vi "Starter Kit 2.0 Custom RT Host.vi"() -> ()   [LabVIEW 2021]
doc: "This VI shows how to use hardware abstracted sensor drivers with a custom FPGA VI to control a Starter Kit robot. This VI runs on the RT host. The main FPGA VI must be compiled before this host VI can be run."
uses:
  <vilib>/rvi/interface/nirviOpenFPGA/nirviOpenFPGA.xnode
  <instrlib>/DC Motor Controller/HAIOL/DC Motor Controller.lvclass
  <vilib>/rvi/interface/nirviCloseFPGA/nirviCloseFPGA.xnode
  <vilib>/rvi/interface/nirviReadWriteControl/nirviReadWriteControl.xnode
  <vilib>/robotics/Utilities/RPM to Radians per Second (Scalar).vi
  <vilib>/robotics/Utilities/Radians per Second to RPM (Scalar).vi
  <vilib>/Utility/AngleManip/NI_AngleManipulation.lvlib
  <vilib>/rvi/interface/Simulation/niFpgaSimulationCallBeginRW.vi
  <vilib>/rvi/errors/niLvFpgaAdjustHostInterfaceError.vi
  <vilib>/Platform/TimedLoop/XDataNode/XDataNode.xnode
  <vilib>/Platform/TimedLoop/XDataNode/nitl_modes.ctl
  <vilib>/Platform/TimedLoop/XDataNode/XDNodeRunTimeDep.lvlib
  <vilib>/Platform/TimedLoop/XDataNode/wakeup.ctl
  <vilib>/Platform/TimedLoop/XDataNode/timing_clust.ctl
  <vilib>/Utility/error.llb/Error Cluster From Error Code.vi
  <instrlib>/Hitec HS400 Series/HAIOL/Hitec HS400 Series.lvclass
  <instrlib>/Parallax PING)))/HAIOL/Parallax PING))).lvclass
  <vilib>/Utility/AngleManip/Degrees to Radians (Scalar DBL).vi
  FPGA Bitfiles/MintaDaNIrobotho_FPGATarget_StarterKit2.0Cus_29373616.lvbitx
  NiFpgaLv.dll
  <vilib>/FPGAPlugInAG/Dynamic/niLvFpga_Close_Dynamic.vi
  <vilib>/FPGAPlugInAG/sbRIO-9632/niLvFpga_Open_sbRIO-9632.vi
  <vilib>/rvi/interface/common/dynamic/niFpgaDynamicAddResources.vi
panel:
  out "P(k|k)":dbl
  out "rho(k|k)":dbl
  out "theta error":dbl
  out "theta(i+1)":dbl
  out "y(i+1)":dbl
  out "x(i+1)":dbl
  out "theta(i)":dbl
  out "y(i)":dbl
  out "x(i)":dbl
  out "right wheel dist":dbl
  out "left wheel dist":dbl
  out "CMPS03 angle":sgl(knob) scale=0.0..360.0 scale format="%#_4f"
  in  "stop":bool
  in  "Common":dbl(slide) min=-100.0 max=100.0 step=4.0 scale=-100.0..100.0
  in  "Diff":dbl(slide) min=-100.0 max=100.0 step=4.0 scale=-100.0..100.0
  out "ccw motor velocities":cluster{"Left":dbl, dbl, "Right":dbl, dbl}(graph)
  in  "sensor motor angle":dbl(slide) caption="Sensor Motor Angle (degrees)" scale=90.0..-90.0
  out "PING))) Sensor Distance (m)":dbl(graph)
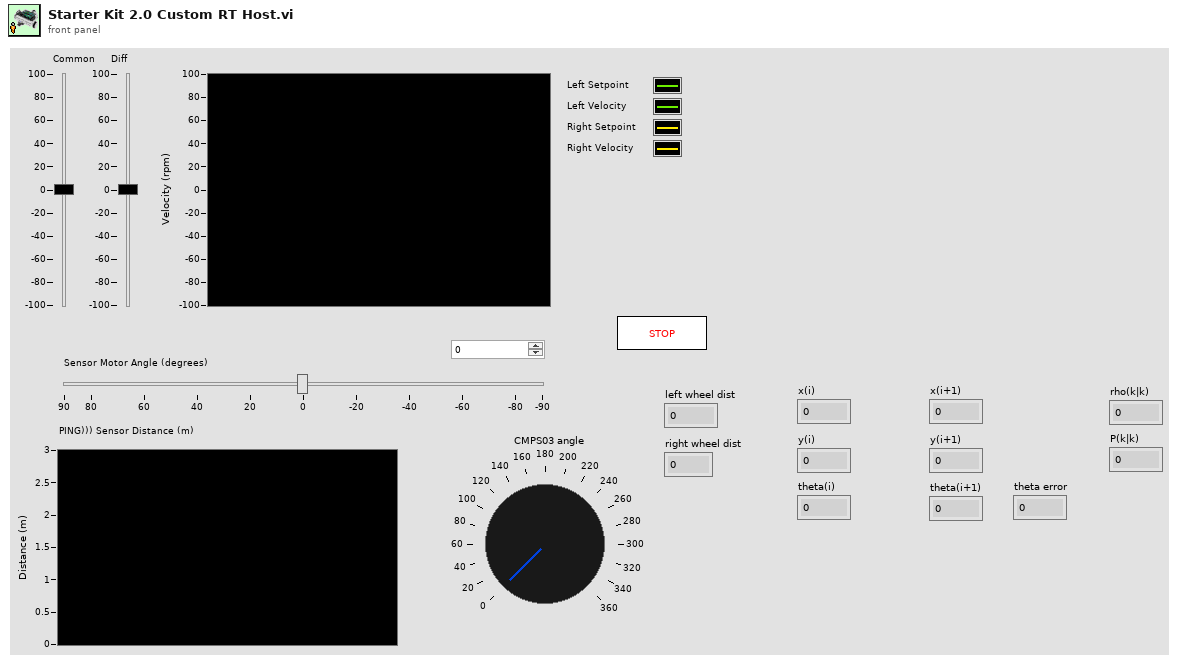
[diagram p1: front panel]
types:
  T1 = typedef "XDNodeRunTimeDep.lvlib/timing_clust.ctl" = cluster{"Expected End [f-1]":u64, "Actual End [f-1]":u64, "Finished Late? [f-1]":bool, "Expected End [i-1]":u64, "Actual End [i-1]":u64, "Finished Late? [i-1]":bool, "Expected Start [i]":u64, "Actual Start [i]":u64, "Expected Start [f]":u64, "Actual Start [f]":u64, "Source Name":string, "Structure Name":string, "Period":i64, "Deadline":i64, "Offset":i64, "Start":i64, "Priority":i32, "Timeout":i32, "Mode":T2, "Wakeup Reason":T3, "Error":errorcluster, "Source Type":string, "Secondary Source Type":string, "Global End Time":u64, "Global Start Time":u64, "Frame Duration":u64, "Iteration Duration":u64, "Assigned CPU":i32, "I/O Scan Engine Mode":u32}
  T2 = typedef "XDNodeRunTimeDep.lvlib/nitl_modes.ctl" = enum32{"No Change", "Process missed periods, maintain original phase", "Discard missed periods, maintain original phase", "Process missed periods, ignore original phase", "Discard missed periods, ignore original phase"}
  T3 = typedef "XDNodeRunTimeDep.lvlib/wakeup.ctl" = enum32{"Normal", "Aborted", "Asynchronous wakeup", "Timing source error", "Timed loop error", "Timeout"}
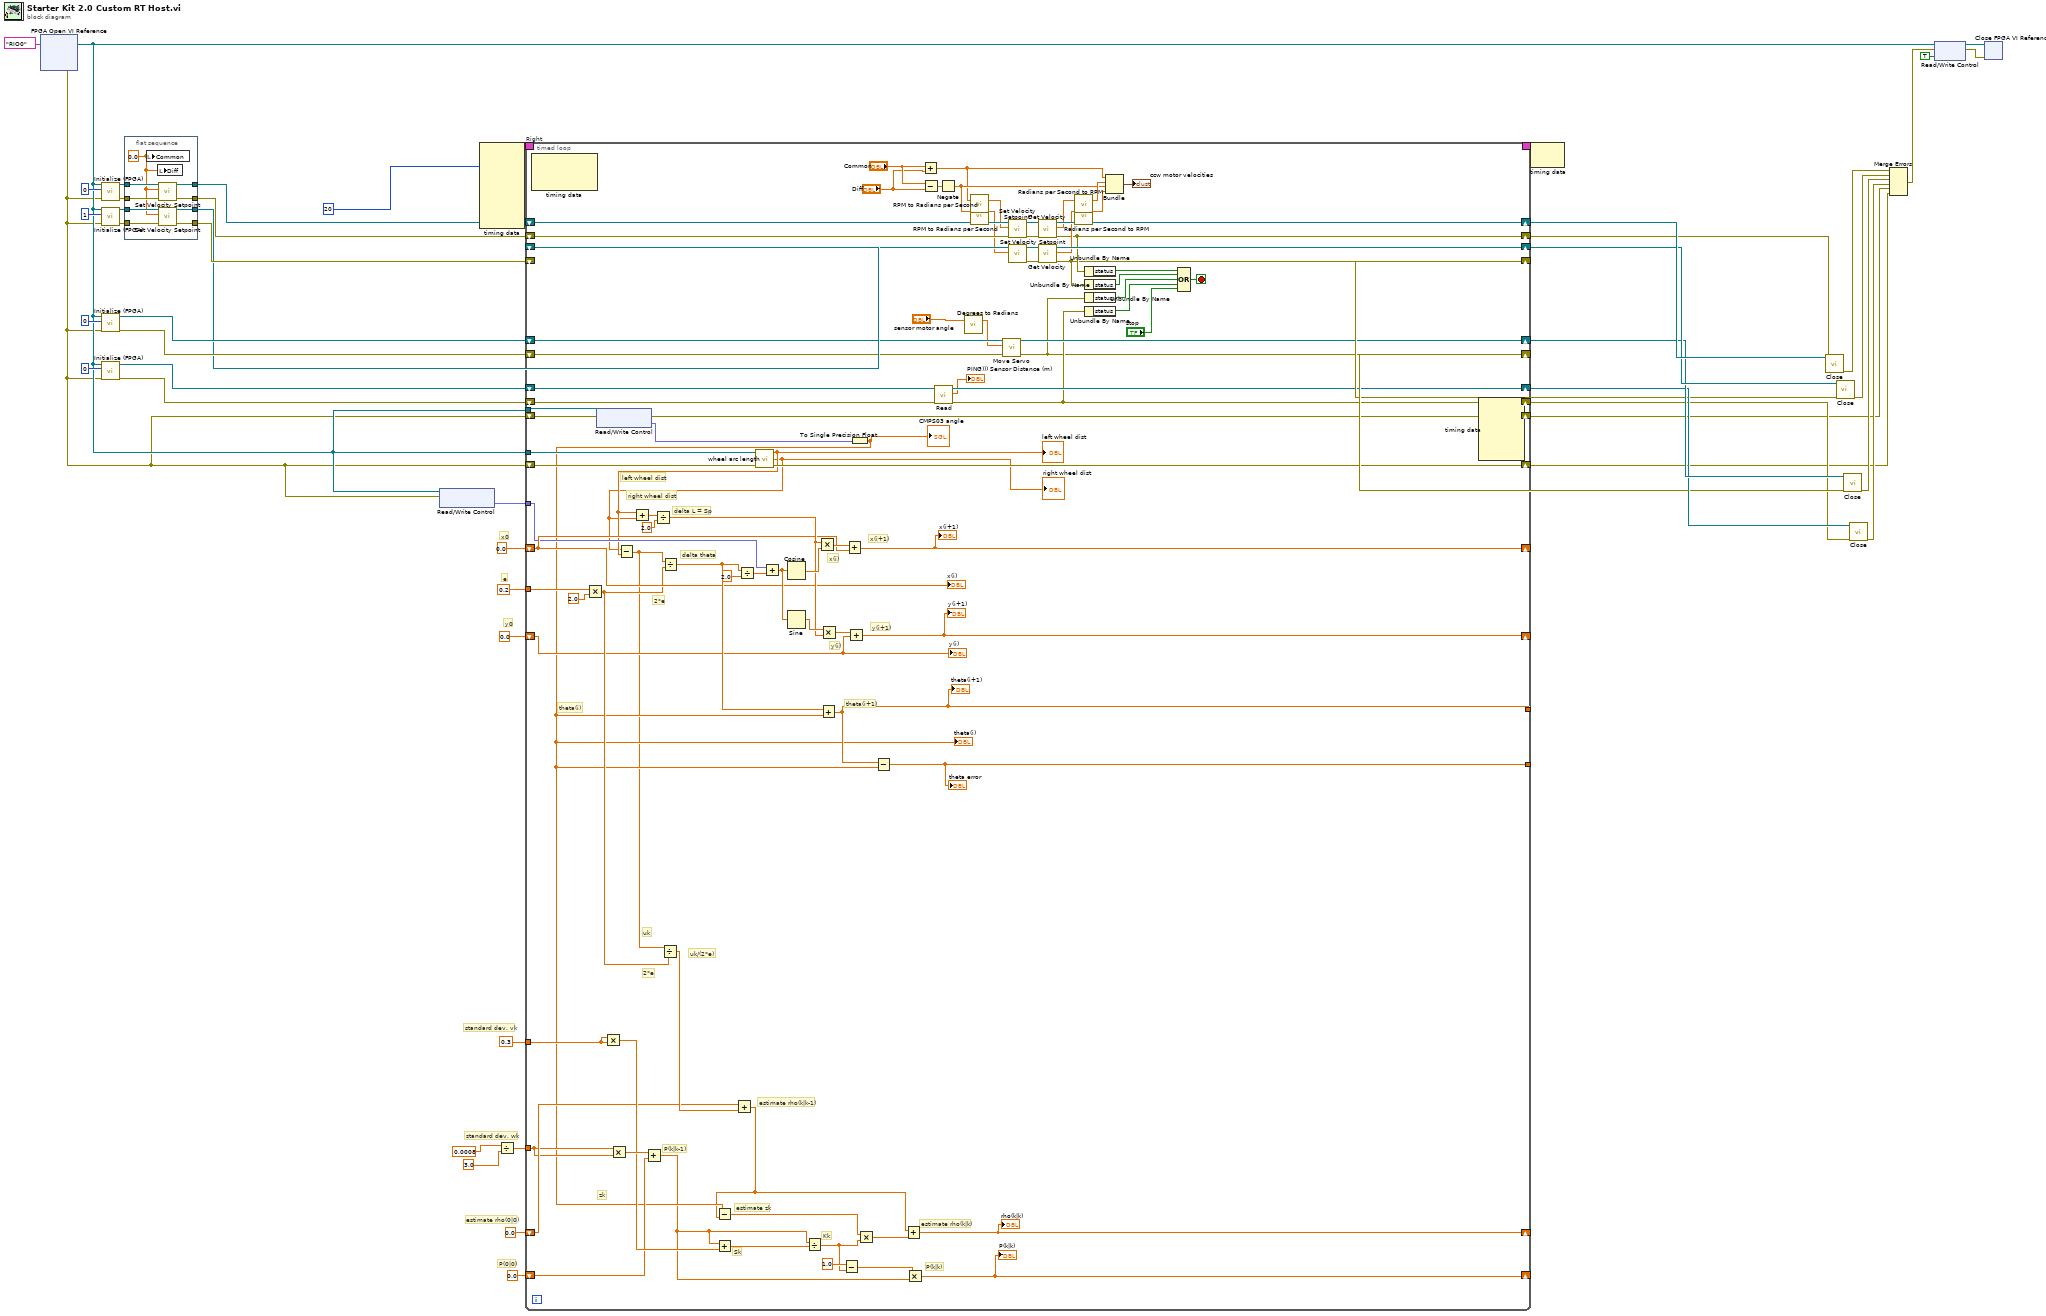
[diagram p0: block diagram]
diagram:
  # "standard dev. vk"
  # "standard dev. wk"
  # "P(0|0)"
  # "estimate rho(0|0)"
  # "y0"
  # "x0"
  # "e"
  n1 = xnode "FPGA Open VI Reference"("resource name"=tag "RIO0") -> ("FPGA VI Reference Out"=w9:refnum<k20>, "error out"=w8:errorcluster)  [unwired: 1 in]
  n2 = call <instrlib>:"Initialize (FPGA).vi"("error in (no error)"=w8, "Actuator ID (0)"=0, "FPGA VI Reference"=w9) -> ("error out"=w24:errorcluster, "DC Motor Controller out"=w26:refnum<class "DC Motor Controller.lvclass">)  [unwired: 7 in]
  n3 = call <instrlib>:"Initialize (FPGA).vi"("error in (no error)"=w8, "Actuator ID (0)"=1, "FPGA VI Reference"=w9) -> ("error out"=w21:errorcluster, "DC Motor Controller out"=w22:refnum<class "DC Motor Controller.lvclass">)  [unwired: 7 in]
  n4 = call <instrlib>:"Initialize (FPGA).vi"("error in (no error)"=w8, "Actuator ID (0)"=0, "FPGA VI Reference"=w9) -> ("error out"=w36:errorcluster, "Hitec HS400 Series out"=w47:refnum<class "Hitec HS400 Series.lvclass">)  [unwired: 7 in]
  n5 = call <instrlib>:"Initialize (FPGA).vi"("error in (no error)"=w8, "Sensor ID (0)"=0, "FPGA VI Reference"=w9) -> ("error out"=w35:errorcluster, "Parallax PING))) out"=w48:refnum<class "Parallax PING))).lvclass">)  [unwired: 7 in]
  n6 = flat-sequence {
    tunnel: w26 -> [w59]
    tunnel: [w58] -> w25
    tunnel: w24 -> [w57]
    tunnel: [w56] -> w23
    tunnel: w22 -> [w55]
    tunnel: [w54] -> w14
    tunnel: w21 -> [w53]
    tunnel: [w52] -> w20
    frame #0 {
      w51 = 0.0 ("CCW Velocity (0 rad/s)")
      n7 = local write "Common"(w51) -> ()
      n8 = local write "Diff"(w51) -> ()
      n9 = call-dynamic "Set Velocity Setpoint.vi"("error in (no error)"=w57, "CCW Velocity (0 rad/s)"=w51, "DC Motor Controller in"=w59) -> ("error out"=w56:errorcluster, "DC Motor Controller out"=w58:refnum<class "DC Motor Controller.lvclass">)  [unwired: 7 in]
      n10 = call-dynamic "Set Velocity Setpoint.vi"("error in (no error)"=w53, "CCW Velocity (0 rad/s)"=w51, "DC Motor Controller in"=w55) -> ("error out"=w52:errorcluster, "DC Motor Controller out"=w54:refnum<class "DC Motor Controller.lvclass">)  [unwired: 7 in]
    }
  }
  n11 = xnode ("Read/Write Control")("FPGA VI Reference In"=w9, "error in"=w8) -> ("CMPS03 angle"=w7:fxp<+,20,16>)  [unwired: 2 out]
  n12 = node-c288(i64 20 ("Period")) -> (w17:T1)  [unwired: 7 in]
  n13 = Divide(x=0.0008, y=3.0) -> (x/y=w4:dbl)
  n14 = timed-loop "Right" {
    shift-right: [w138] -> w43
    shift-left: w48 -> [w148]
    shift-right: [w135] -> w44
    shift-left: w47 -> [w147]
    shift-right: [w144] -> w46
    shift-left: w25 -> [w146]
    shift-right: [w141] -> w45
    shift-left: w14 -> [w143]
    shift-right: [w129] -> w37
    shift-left: w23 -> [w140]
    shift-right: [w128] -> w32
    shift-left: w20 -> [_]
    shift-right: [w126] -> w34
    shift-left: w36 -> [w136]
    shift-right: [w127] -> w33
    shift-left: w35 -> [w137]
    tunnel: w9 -> [w68]
    shift-right: [w114] -> w19
    shift-left: w8 -> [w115]
    tunnel: w9 -> [w113]
    shift-right: [w105] -> w18
    shift-left: w8 -> [w107]
    timing: w17 -> [_]
    timing-out: [_] -> w16
    tunnel: 0.2 -> [w101]
    shift-right: [w67] -> _
    shift-left: 0.0 -> [w90]
    shift-right: [w89] -> _
    shift-left: 0.0 -> [w66]
    tunnel: [w88] -> _
    tunnel: w7 -> [w73]
    tunnel: [w87] -> _
    tunnel: w4 -> [w71]
    tunnel: 0.3 ("standard deviation") -> [w82]
    shift-right: [w70] -> _
    shift-left: 0.0 -> [w78]
    shift-right: [w69] -> _
    shift-left: 0.0 -> [w74]
    stop <- w121 stop-if-true
    # "left wheel dist"
    # "right wheel dist"
    # "2*e"
    # "theta(i)"
    # "zk"
    # "uk/(2*e)"
    # "2*e"
    # "P(k|k)"
    # "estimate rho(k|k)"
    # "Kk"
    # "Sk"
    # "P(k|k-1)"
    # "estimate rho(k|k-1)"
    # "estimate zk"
    # "uk"
    # "theta(i+1)"
    # "y(i)"
    # "y(i+1)"
    # "x(i)"
    # "x(i+1)"
    # "delta theta"
    # "delta L = Sp"
    n15 = node-c288() -> ()  [unwired: 1 in, 3 out]
    n16 = Multiply(x=w101, y=2.0) -> (x*y=w86:dbl)
    n17 = xnode ("Read/Write Control")("FPGA VI Reference In"=w68, "error in"=w115) -> ("error out"=w114:errorcluster, "CMPS03 angle"=w72:fxp<+,20,16>)  [unwired: 1 out]
    n18 = Multiply(x=w82, y=w82) -> (x*y=w83:dbl)
    n19 = Multiply(x=w71, y=w71) -> (x*y=w84:dbl)
    n20 = Add(x=w84, y=w74) -> (x+y=w61:dbl)
    n21 = Add(x=w61, y=w83) -> (x+y=w81:dbl)
    n22 = call "wheel arc length.vi"("error in"=w107, "FPGA VI Reference In"=w113) -> ("error out"=w105:errorcluster, "Right arc in m"=w62:dbl, "Left arc in m"=w64:dbl)  [unwired: 1 in]
    "left wheel dist" <- w64
    "right wheel dist" <- w62
    n23 = Subtract(x=w62, y=w64) -> (x-y=w63:dbl)
    n24 = Add(x=w64, y=w62) -> (x+y=w103:dbl)
    n25 = Divide(x=w103, y=2.0) -> (x/y=w92:dbl)
    n26 = Divide(x=w63, y=w86) -> (x/y=w85:dbl)
    n27 = Divide(x=w63, y=w86) -> (x/y=w91:dbl)
    n28 = Add(x=w78, y=w85) -> (x+y=w60:dbl)
    n29 = Divide(x=w91, y=2.0) -> (x/y=w99:dbl)
    n30 = Add(x=w73, y=w99) -> (x+y=w95:dbl)
    n31 = Cosine(x=w95) -> (cos(x)=w97:dbl)
    n32 = Sine(x=w95) -> (sin(x)=w93:dbl)
    n33 = Divide(x=w61, y=w81) -> (x/y=w76:dbl)
    n34 = Multiply(x=w92, y=w97) -> (x*y=w96:dbl)
    n35 = Multiply(x=w93, y=w92) -> (x*y=w94:dbl)
    n36 = Subtract(x=1.0, y=w76) -> (x-y=w75:dbl)
    n37 = Add(x=w96, y=w90) -> (x+y=w67:dbl)
    "x(i+1)" <- w67
    n38 = Add(x=w94, y=w66) -> (x+y=w89:dbl)
    "y(i+1)" <- w89
    n39 = To Single Precision Float(number=w72) -> (single precision float=w65:sgl)
    "CMPS03 angle" <- w65
    "theta(i)" <- w65
    n40 = Subtract(x=w65, y=w60) -> (x-y=w80:dbl)
    n41 = Add(x=w91, y=w65) -> (x+y=w88:dbl)
    "theta(i+1)" <- w88
    n42 = Multiply(x=w80, y=w76) -> (x*y=w79:dbl)
    n43 = Subtract(x=w88, y=w65) -> (x-y=w87:dbl)
    "theta error" <- w87
    n44 = Add(x=w60, y=w79) -> (x+y=w70:dbl)
    "rho(k|k)" <- w70
    n45 = Multiply(x=w75, y=w61) -> (x*y=w69:dbl)
    "P(k|k)" <- w69
    n46 = Add(x="Common", y="Diff") -> (x+y=w109:dbl)
    n47 = Subtract(x="Common", y="Diff") -> (x-y=w111:dbl)
    n48 = call-dynamic "Read.vi"("error in (no error)"=w137, "Parallax PING))) in"=w148) -> ("error out"=w127:errorcluster, "Distance (m)"=→"PING))) Sensor Distance (m)":dbl, "Parallax PING))) out"=w138:refnum<class "Parallax PING))).lvclass">)  [unwired: 6 in, 1 out]
    n49 = Negate(x=w111) -> (-x=w112:dbl)
    n50 = call-poly <vilib>:"Degrees to Radians.vi"("angle (deg)"="sensor motor angle") -> ("angle (rad)"=w117:dbl)  [unwired: 2 in]
    n51 = call-poly <vilib>:"RPM to Radians per Second.vi"("rpm"=w109) -> ("radians per second"=w130:dbl)  [unwired: 2 in]
    n52 = call-poly <vilib>:"RPM to Radians per Second.vi"("rpm"=w112) -> ("radians per second"=w131:dbl)  [unwired: 2 in]
    n53 = call-dynamic "Move Servo.vi"("error in (no error)"=w136, "CCW Position (0.0 rad)"=w117, "Hitec HS400 Series in"=w147) -> ("error out"=w126:errorcluster, "Hitec HS400 Series out"=w135:refnum<class "Hitec HS400 Series.lvclass">)  [unwired: 7 in]
    n54 = call-dynamic "Set Velocity Setpoint.vi"("error in (no error)"=w140, "CCW Velocity (0 rad/s)"=w130, "DC Motor Controller in"=w146) -> ("error out"=w139:errorcluster, "DC Motor Controller out"=w145:refnum<class "DC Motor Controller.lvclass">)  [unwired: 7 in]
    n55 = call-dynamic "Set Velocity Setpoint.vi"("CCW Velocity (0 rad/s)"=w131, "DC Motor Controller in"=w143) -> ("error out"=w134:errorcluster, "DC Motor Controller out"=w142:refnum<class "DC Motor Controller.lvclass">)  [unwired: 8 in]
    n56 = call-dynamic "Get Velocity.vi"("error in (no error)"=w139, "DC Motor Controller in"=w145) -> ("error out"=w129:errorcluster, "CCW Velocity (rad/s)"=w133:dbl, "DC Motor Controller out"=w144:refnum<class "DC Motor Controller.lvclass">)  [unwired: 7 in]
    n57 = call-dynamic "Get Velocity.vi"("error in (no error)"=w134, "DC Motor Controller in"=w142) -> ("error out"=w128:errorcluster, "CCW Velocity (rad/s)"=w132:dbl, "DC Motor Controller out"=w141:refnum<class "DC Motor Controller.lvclass">)  [unwired: 7 in]
    n58 = call-poly <vilib>:"Radians per Second to RPM.vi"("radians per second"=w133) -> ("rpm"=w120:dbl)  [unwired: 2 in]
    n59 = call-poly <vilib>:"Radians per Second to RPM.vi"("radians per second"=w132) -> ("rpm"=w119:dbl)  [unwired: 2 in]
    n60 = Unbundle By Name(w129) -> ("status"=w125:bool)
    n61 = Unbundle By Name(w128) -> ("status"=w124:bool)
    n62 = Unbundle By Name(w126) -> ("status"=w123:bool)
    n63 = Unbundle By Name(w127) -> ("status"=w122:bool)
    n64 = Bundle(w109, "rpm"=w120, w112, "rpm"=w119) -> (→"ccw motor velocities":cluster{dbl, "rpm":dbl, dbl, "rpm":dbl})  [unwired: 1 in]
    n65 = Compound Arithmetic op=OR(w125, w124, w123, w122, "stop") -> (w121:bool)
    n66 = node-c288() -> ()  [unwired: 6 in, 1 out]
    "y(i)" <- w66
    "x(i)" <- w90
  }
  n67 = node-c288(w16) -> ()  [unwired: 1 out]
  n68 = call-dynamic "Close.vi"("error in (no error)"=w37, "DC Motor Controller in"=w46) -> ("error out"=w31:errorcluster)  [unwired: 9 in]
  n69 = call-dynamic "Close.vi"("error in (no error)"=w32, "DC Motor Controller in"=w45) -> ("error out"=w30:errorcluster)  [unwired: 9 in]
  n70 = call-dynamic "Close.vi"("error in (no error)"=w34, "Hitec HS400 Series in"=w44) -> ("error out"=w29:errorcluster)  [unwired: 9 in]
  n71 = call-dynamic "Close.vi"("error in (no error)"=w33, "Parallax PING))) in"=w43) -> ("error out"=w28:errorcluster)  [unwired: 9 in]
  n72 = Merge Errors(w31, w30, w29, w28, w19, w18) -> (w27:errorcluster)
  n73 = xnode "Read/Write Control"("FPGA VI Reference In"=w9, "error in"=w27, "stop"=TRUE) -> ("FPGA VI Reference Out"=w40:refnum<k20>, "error out"=w39:errorcluster)
  n74 = xnode "Close FPGA VI Reference"("FPGA VI Reference In"=w40, "error in"=w39) -> ()  [unwired: 1 out]
